vi "Conveyor Calibrations.vi"() -> ()   [LabVIEW 2016]
panel:
  in  "Conveyor Calibrations File Location":path=path "C:/ni-rt/startup/ConveyorCalibrations.txt"
  out "Conveyor Normal Drive Speed (throttle)":dbl
  out "Conveyor Reset Speed (throttle)":dbl
  out "Conveyor Manual Reverse Speed (throttle)":dbl
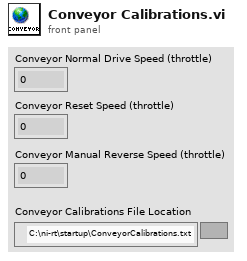
[diagram p1: front panel]
diagram:
